vi "lab1_variant_01.vi"(11 "X":dbl) -> (2 "Z(x)":dbl)   [LabVIEW 2026]
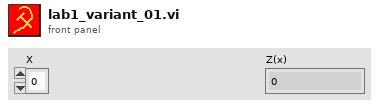
[diagram p1: front panel]
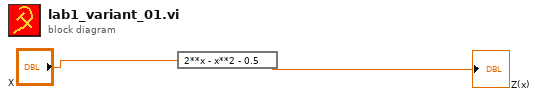
[diagram p0: block diagram]
diagram:
  n1 = expression code="2**x - x**2 - 0.5"("X") -> (→"Z(x)":dbl)
